vi "ADAM6018.vi"(4 "Scan Period":dbl format="%.2f", 5 "Previous Scan Value":dbl format="%.2f", 6 "Present scan array":dbl[](array[numeric]) format="%.2f", 7 "Value to Output":dbl format="%.2f", 8 "Ch Description":T1={"Ch Name"="", "Type"="", "Function"=enum."Analogue Input", "Ch State"=enum."On", "Calibration type"="", "A"=0.0, "B"=0.0, "C"=0.0, "D"=0.0, "Comments"="", "Address"={"Main"=0, "Ch."=0, "Sub"=0, "Port Name"="192.168.120.110"}, "String"="", "Duty"=65535} {"Duty" format="%016b"; "D" format="%#_5g"; "C" format="%#_5g"; "B" format="%#_5g"; "A" format="%#_5g"}, 9 "Ch names":string[](array[string])) -> (0 "Scan comment":string, 1 "Output":dbl format="%.3f", 3 "HelpText":string="Add helpful help text here!")   [LabVIEW 2022 SP3]
uses:
  ADAM Client/Sub VIs/ADAM Controls/Ch_description_ADAM.ctl
  ADAM Client/Sub VIs/ADAM Controls/Module_type_ADAM.ctl
  ADAM Client/Sub VIs/ADAM Controls/Function_ADAM.ctl
  ADAM Client/Sub VIs/ADAM Controls/Channel_State.ctl
  ADAM Client/Sub VIs/ADAM Controls/Calib_type_ADAM.ctl
  ADAM Client/Sub VIs/ADAM Controls/Address.ctl
  <vilib>/Utility/error.llb/DialogType.ctl
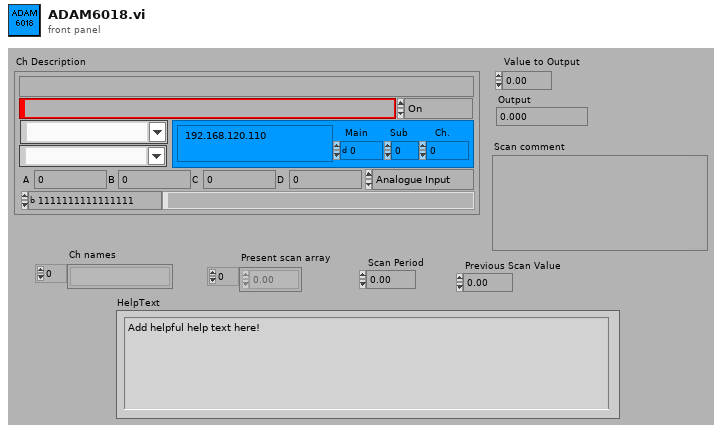
[diagram p1: front panel]
types:
  T1 = typedef "Ch_description_ADAM.ctl" = cluster{"Ch Name":string, "Type":T2, "Function":T3, "Ch State":T4, "Calibration type":T5, "A":dbl, "B":dbl, "C":dbl, "D":dbl, "Comments":string, "Address":T6, "String":string, "Duty":u16}
  T2 = typedef "Module_type_ADAM.ctl" = string
  T3 = typedef "Function_ADAM.ctl" = enum16{"Analogue Input", "Digital Input", "Event counter", "Event rate", "Analogue Output", "Digital Output", "Relay Output"}
  T4 = typedef "Channel_State.ctl" = enum16{"On", "Off", "Always On", "Always Off"}
  T5 = typedef "Calib_type_ADAM.ctl" = string
  T6 = typedef "Address.ctl" = cluster{"Main":i32, "Ch.":i32, "Sub":i32, "Port Name":string}
  T7 = typedef "DialogType.ctl" = u16
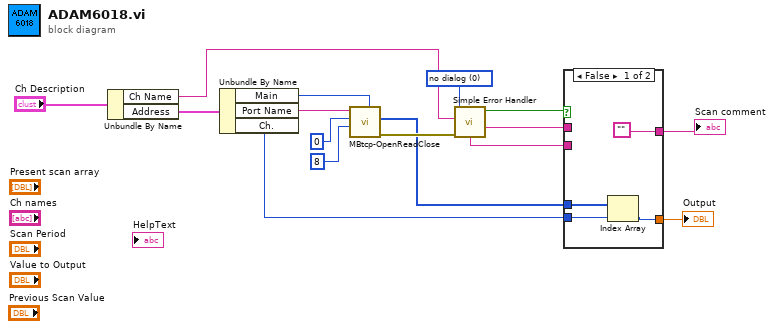
[diagram p0: block diagram]
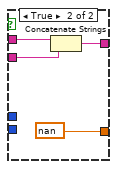
[diagram p2: hidden frame]
diagram:
  w15 = T7 0 items=["no dialog", "OK message", "continue or stop message", "OK message + warnings", "continue/stop + warnings"] ("type of dialog (OK msg:1)")
  n1 = Unbundle By Name("Ch Description") -> ("Ch Name"=w10:string, "Address"=w12:T6)
  n2 = Unbundle By Name(w12) -> ("Main"=w1:i32, "Port Name"=w6:string, "Ch."=w11:i32)
  n3 = call "MBtcp-OpenReadClose.vi"("Slave ID"=w1, "nRegisters"=u16 8, "RegisterAddr"=u16 0, "IP Address(:port)"=w6) -> ("error out"=w5:errorcluster, "16bitValues"=w4:u16[])  [unwired: 5 in, 1 out]
  n4 = call <vilib>:"Simple Error Handler.vi"("error source (\" \")"=w10, "type of dialog (OK msg:1)"=w15, "error in (no error)"=w5) -> ("error?"=w9:bool, "source out"=w13:string, "message"=w14:string)  [unwired: 4 out]
  n5 = case shown="False" w9 {
    tunnel: w14 -> [_ w22]
    tunnel: w13 -> [_ w23]
    tunnel: w11 -> [w20 _]
    tunnel: ["" w21] -> w8
    tunnel: [w19 nan ("t")] -> w7
    tunnel: w4 -> [w17 _]
    frame False {
      n6 = Index Array(array=w17, index=w20) -> (element=w19:u16)
    }
    frame True {
      n7 = Concatenate Strings(w23, w22) -> (w21:string)
    }
  }
  "Output" <- w7
  "Scan comment" <- w8
